vi "SoloCamera.vi"() -> ()   [LabVIEW 2019]
panel:
  in  "Press to take":bool=TRUE
  in  "Camera Name":refnum<k21>="cam0" caption="IMAQdx Session"
  out "Current image":T1(plugin-control)
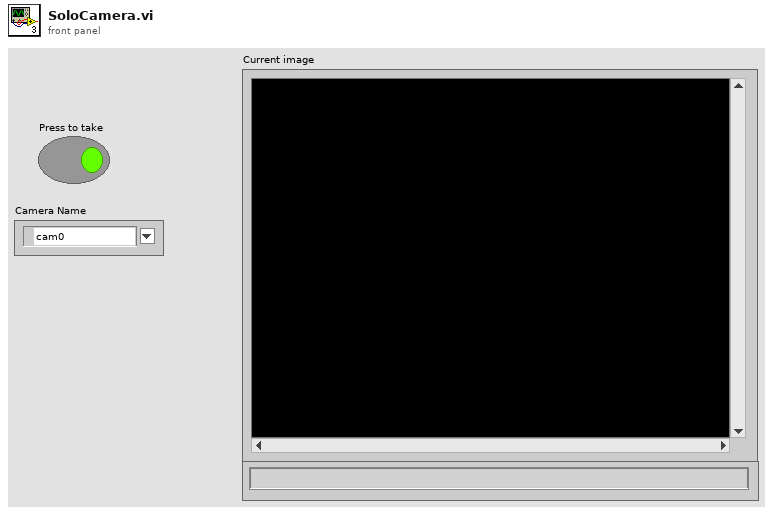
[diagram p1: front panel]
types:
  T1 = typedef "IMAQ Image.ctl" = refnum<image>
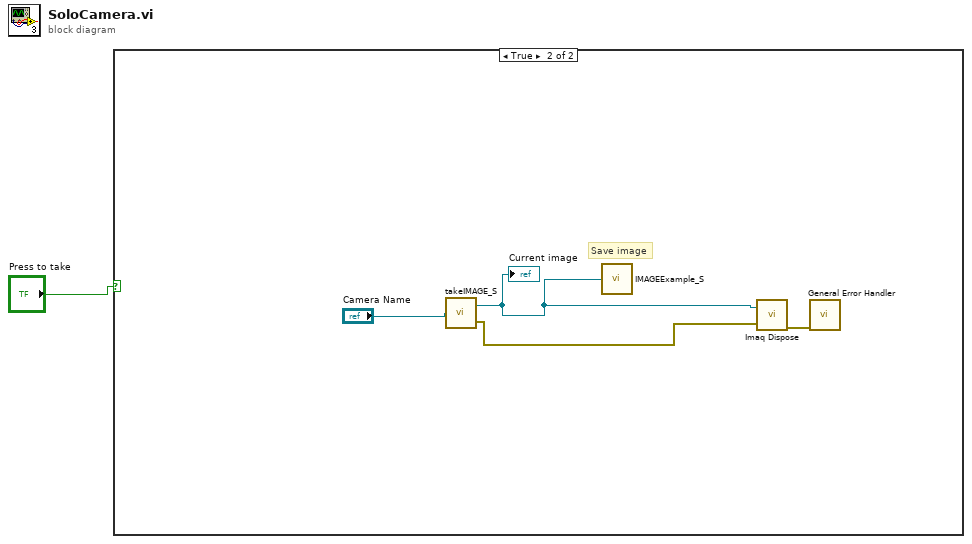
[diagram p0: block diagram]
diagram:
  n1 = case shown="True" "Press to take" {
    frame False {
    }
    frame True {
      # "Save image"
      n2 = call "takeIMAGE_S.vi"("Camera Name"="Camera Name") -> ("Current image"=w3:T1, "error in (no error)"=w2:errorcluster)
      "Current image" <- w3
      n3 = call "IMAGEExample_S.vi"("Image"=w3) -> ()  [unwired: 1 out]
      n4 = call "Imaq Dispose"("Image"=w3, "error in (no error)"=w2) -> ("error out"=w4:errorcluster)  [unwired: 4 in]
      n5 = call <vilib>:"General Error Handler.vi"("error in (no error)"=w4) -> ()  [unwired: 2 in, 13 out]
    }
  }
